vi "InlineCustomDeviceDriverVIModelInterface_Good.vi"(7 "Operation":T1, 11 "Device Reference in":T2 format="%.0x") -> (0 "Error Code":i32)   [LabVIEW 2015]
uses:
  <vilib>/NI Veristand/Custom Device API/Custom Device Item Ref.ctl
  <vilib>/NI Veristand/Custom Device API/Model Interface Driver VI Operation.ctl
  <vilib>/NI Veristand/Custom Device API/Custom Device Channel Type.ctl
  <vilib>/NI Veristand/Custom Device API/Data Reference.ctl
  <vilib>/NI Veristand/Custom Device API/Data Access Type.ctl
  <vilib>/NI Veristand/Custom Device API/Global Data Refs.vi
  <vilib>/NI Veristand/Custom Device API/Custom Device API.lvlib
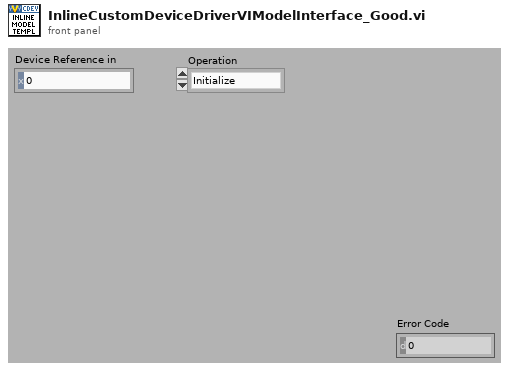
[diagram p1: front panel]
types:
  T1 = typedef "Custom Device API.lvlib/Model Interface Driver VI Operation.ctl" = enum16{"Initialize", "Start", "Execute Model", "Close"}
  T2 = typedef "Custom Device API.lvlib/Custom Device Item Ref.ctl" = u64
  T3 = typedef "Custom Device API.lvlib/Data Reference.ctl" = i32
  T4 = cluster{"Input Values":dbl[], "Input Refs":T3[], "Output Values":dbl[], "Output Refs":T3[]}
  T5 = typedef "Custom Device API.lvlib/Custom Device Channel Type.ctl" = enum16{"Input", "Output"}
  T6 = typedef "Custom Device API.lvlib/Data Access Type.ctl" = enum16{"Read", "Write"}
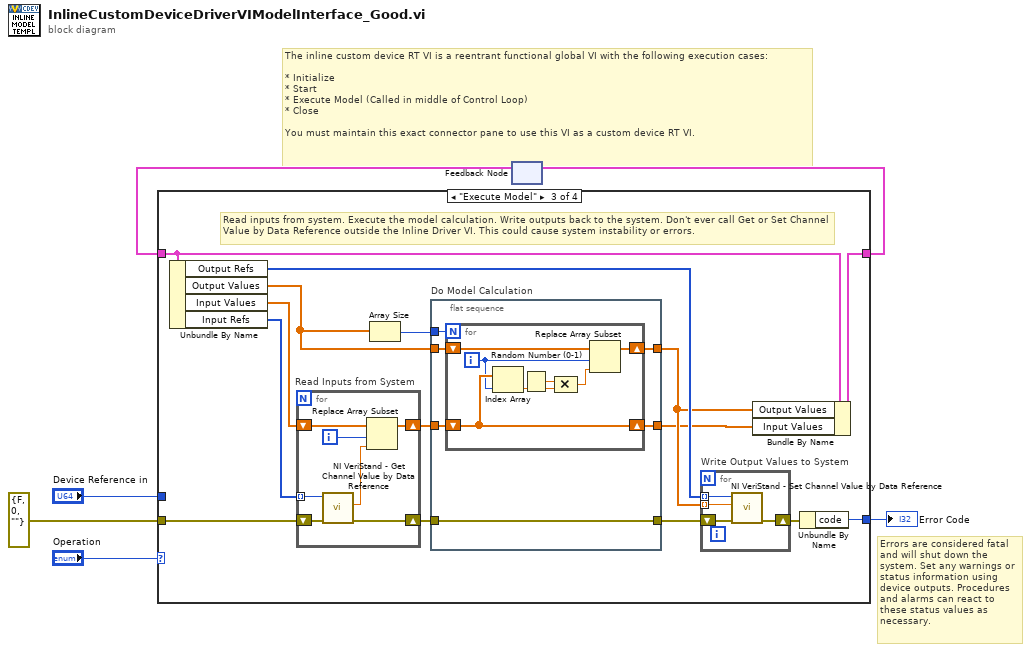
[diagram p0: block diagram]
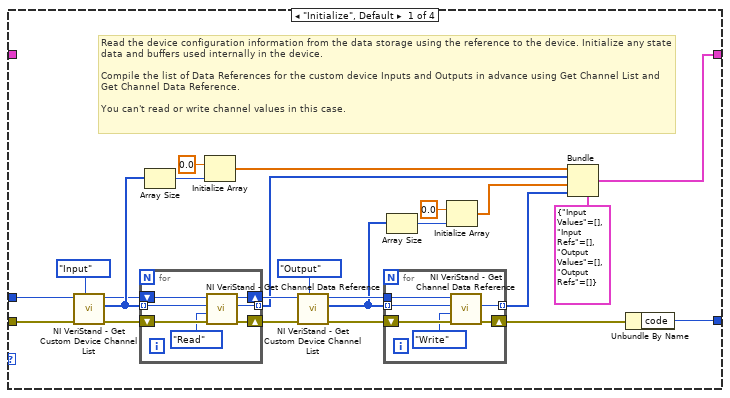
[diagram p2: hidden frame]
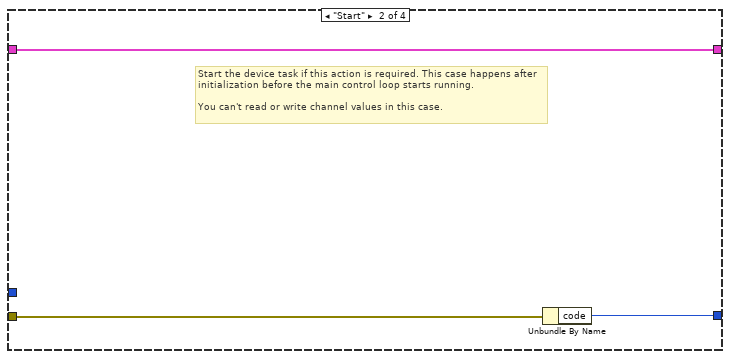
[diagram p3: hidden frame]
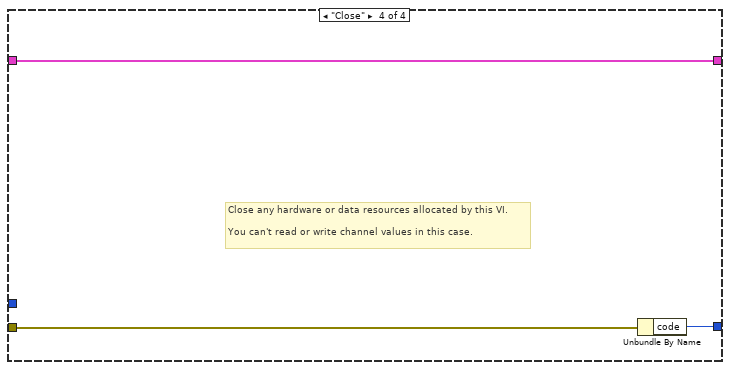
[diagram p4: hidden frame]
diagram:
  # "Errors are considered fatal and will shut down the system. Set any warnings or status information using device outputs. Procedures and alarms can react to these status values as necessary."
  # "The inline custom device RT VI is a reentrant functional global VI with the following execution cases:\n\n* Initialize\n* Start\n* Execute Model (Called in middle of Control Loop)\n* Close\n\nYou must maintain this exact connector pane to use this VI as a custom device RT VI."
  n1 = feedback #1() -> (w4:T4)  [unwired: 1 out]
  n2 = case shown="\"Execute Model\"" "Operation" {
    tunnel: [w9 w46 w54 w88] -> w5
    tunnel: w4 -> [_ w46 w55 w88]
    tunnel: "Device Reference in" -> [w10 _ _ _]
    tunnel: [w8 w44 w50 w87] -> w2
    tunnel: errorcluster {"status"=FALSE, "code"=0, "source"=""} ("error in (no error)") -> [w7 w45 w59 w86]
    frame "Initialize", Default {
      # "Read the device configuration information from the data storage using the reference to the device. Initialize any state data and buffers used internally in the device.\n\nCompile the list of Data References for the custom device Inputs and Outputs in advance using Get Channel List and Get Channel Data Reference.\n\nYou can't read or write channel values in this case."
      n3 = call <vilib>:"NI VeriStand - Get Custom Device Channel List.vi"("Channel Type"=Custom_Device_Channel_Type."Input", "error in (no error)"=w7, "Device Ref in"=w10) -> ("error out"=w16:errorcluster, "Specified Channel Ref List"=w17:T2[], "Device Ref out"=w15:T2)  [unwired: 6 out]
      n4 = for {
        shift-right: [w38] -> w29
        shift-left: w15 -> [w42]
        tunnel: w17 -> [w41] mode=indexing
        shift-right: [w39] -> w20
        shift-left: w16 -> [w43]
        tunnel: [w37] -> w21 mode=indexing
        n5 = call <vilib>:"NI VeriStand - Get Channel Data Reference.vi"("error in (no error)"=w43, "Access"=Data_Access_Type."Read", "Channel Ref in"=w41, "Device Ref in"=w42) -> ("error out"=w39:errorcluster, "Channel Data Reference"=w37:T3, "Device Ref out"=w38:T2)  [unwired: 5 out]
      }
      n6 = Array Size(array=w17) -> (size(s)=w12:i32)
      n7 = Initialize Array(0.0 ("element"), w12) -> (w11:dbl[])
      n8 = call <vilib>:"NI VeriStand - Get Custom Device Channel List.vi"("Channel Type"=Custom_Device_Channel_Type."Output", "error in (no error)"=w20, "Device Ref in"=w29) -> ("error out"=w18:errorcluster, "Specified Channel Ref List"=w24:T2[], "Device Ref out"=w30:T2)  [unwired: 6 out]
      n9 = for {
        tunnel: w24 -> [w34] mode=indexing
        shift-right: [w32] -> w27
        shift-left: w18 -> [w36]
        tunnel: [w31] -> w26 mode=indexing
        tunnel: w30 -> [w35]
        n10 = call <vilib>:"NI VeriStand - Get Channel Data Reference.vi"("error in (no error)"=w36, "Access"=Data_Access_Type."Write", "Channel Ref in"=w34, "Device Ref in"=w35) -> ("error out"=w32:errorcluster, "Channel Data Reference"=w31:T3)  [unwired: 6 out]
      }
      n11 = Array Size(array=w24) -> (size(s)=w23:i32)
      n12 = Initialize Array(0.0 ("element"), w23) -> (w25:dbl[])
      n13 = Bundle(cluster=T4 {"Input Values"=[], "Input Refs"=[], "Output Values"=[], "Output Refs"=[]}, "Input Values"=w11, "Input Refs"=w21, "Output Values"=w25, "Output Refs"=w26) -> (w9:T4)
      n14 = Unbundle By Name(w27) -> ("code"=w8:i32)
    }
    frame "Start" {
      # "Start the device task if this action is required. This case happens after initialization before the main control loop starts running.\n\nYou can't read or write channel values in this case."
      n15 = Unbundle By Name(w45) -> ("code"=w44:i32)
    }
    frame "Execute Model" {
      # "Read inputs from system. Execute the model calculation. Write outputs back to the system. Don't ever call Get or Set Channel Value by Data Reference outside the Inline Driver VI. This could cause system instability or errors."
      n16 = Unbundle By Name(w55) -> ("Output Refs"=w53:T3[], "Output Values"=w48:dbl[], "Input Values"=w61:dbl[], "Input Refs"=w60:T3[])
      n17 = for "Read Inputs from System" {
        shift-right: [w79] -> w57
        shift-left: w59 -> [w85]
        tunnel: w60 -> [w84] mode=indexing
        shift-right: [w82] -> w58
        shift-left: w61 -> [w83]
        i -> [w81]
        n18 = call <vilib>:"NI VeriStand - Get Channel Value by Data Reference.vi"("error in (no error)"=w85, "Data Reference in"=w84) -> ("error out"=w79:errorcluster, "Value"=w80:dbl)  [unwired: 8 out]
        n19 = Replace Array Subset(array=w83, new element=w80, index=w81) -> (w82:dbl[])
      }
      n20 = Array Size(array=w48) -> (size(s)=w47:i32)
      n21 = flat-sequence "Do Model Calculation" {
        tunnel: w58 -> [w69]
        tunnel: w57 -> [w71]
        tunnel: w48 -> [w70]
        tunnel: [w68] -> w49
        tunnel: [w67] -> w52
        tunnel: [w71] -> w56
        tunnel: w47 -> [w66]
        frame #0 {
          n22 = for {
            N: w66 -> [_]
            shift-right: [w77] -> w67
            shift-left: w70 -> [w78]
            shift-right: [w74] -> w68
            shift-left: w69 -> [w74]
            i -> [w72]
            n23 = Index Array(array=w74, index=w72) -> (element=w73:dbl)
            n24 = Random Number (0-1)() -> (number: 0 to 1=w76:dbl)
            n25 = Compound Arithmetic op=MULTIPLY(w76, w73) -> (w75:dbl)
            n26 = Replace Array Subset(array=w78, new element=w75, index=w72) -> (w77:dbl[])
          }
        }
      }
      n27 = for "Write Output Values to System" {
        shift-right: [w64] -> w51
        shift-left: w56 -> [w65]
        tunnel: w52 -> [w63] mode=indexing
        tunnel: w53 -> [w62] mode=indexing
        n28 = call <vilib>:"NI VeriStand - Set Channel Value by Data Reference.vi"("error in (no error)"=w65, "Value"=w63, "Data Reference in"=w62) -> ("error out"=w64:errorcluster)  [unwired: 8 out]
      }
      n29 = Bundle By Name(cluster=w55, "Output Values"=w52, "Input Values"=w49) -> (w54:T4)
      n30 = Unbundle By Name(w51) -> ("code"=w50:i32)
    }
    frame "Close" {
      # "Close any hardware or data resources allocated by this VI.\n\nYou can't read or write channel values in this case."
      n31 = Unbundle By Name(w86) -> ("code"=w87:i32)
    }
  }
  "Error Code" <- w2
  n32 = feedback-in #1(w5) -> ()
